vi "NN_Get_Incorrect_Classified_Imgs(GrayScale)_1D.vi"(6 "Test_Data":T2={"Inputs Ref."=variant(refnum<data-value> refnum), "Outputs Ref."=refnum, "Dims_In"=0, "Dataset_Size"=0, "Dims_Out"=0, "Labels"=[], "File Paths"=[]}, 8 "error in (no error)":errorcluster, 10 "Predictions":sgl[][](array[numeric]), 11 "MisClassed_idx":i32[](array[numeric])) -> (0 "error out":errorcluster, 3 "Images(GrayScale)":T1[][](array[typedef])=[[{"image"=array28x28[784 elements], "Truth"=4, "Predicted"=0}, {"image"=array28x28[784 elements], "Truth"=9, "Predicted"=0}, {"image"=array28x28[784 elements], "Truth"=4, "Predicted"=0}, {"image"=array28x28[784 elements], "Truth"=9, "Predicted"=0}, {"image"=array28x28[784 elements], "Truth"=2, "Predicted"=0}, {"image"=array28x28[784 elements], "Truth"=5, "Predicted"=0}, {"image"=array28x28[784 elements], "Truth"=3, "Predicted"=0}, {"image"=array28x28[784 elements], "Truth"=6, "Predicted"=0}, {"image"=array28x28[784 elements], "Truth"=9, "Predicted"=0}, {"image"=array28x28[784 elements], "Truth"=3, "Predicted"=0}], [{"image"=array28x28[784 elements], "Truth"=8, "Predicted"=0}, {"image"=array28x28[784 elements], "Truth"=8, "Predicted"=0}, {"image"=array28x28[784 elements], "Truth"=2, "Predicted"=0}, {"image"=array28x28[784 elements], "Truth"=7, "Predicted"=0}, {"image"=array28x28[784 elements], "Truth"=5, "Predicted"=0}, {"image"=array28x28[784 elements], "Truth"=4, "Predicted"=0}, {"image"=array28x28[784 elements], "Truth"=4, "Predicted"=0}, {"image"=array28x28[784 elements], "Truth"=8, "Predicted"=0}, {"image"=array28x28[784 elements], "Truth"=8, "Predicted"=0}, {"image"=array28x28[784 elements], "Truth"=5, "Predicted"=0}], [{"image"=array28x28[784 elements], "Truth"=5, "Predicted"=0}, {"image"=array28x28[784 elements], "Truth"=6, "Predicted"=0}, {"image"=array28x28[784 elements], "Truth"=7, "Predicted"=0}, {"image"=array28x28[784 elements], "Truth"=4, "Predicted"=0}, {"image"=array28x28[784 elements], "Truth"=3, "Predicted"=0}, {"image"=array28x28[784 elements], "Truth"=7, "Predicted"=0}, {"image"=array28x28[784 elements], "Truth"=6, "Predicted"=0}, {"image"=array28x28[784 elements], "Truth"=9, "Predicted"=0}, {"image"=array28x28[784 elements], "Truth"=2, "Predicted"=0}, {"image"=array28x28[784 elements], "Truth"=7, "Predicted"=0}], [{"image"=array28x28[784 elements], "Truth"=4, "Predicted"=0}, {"image"=array28x28[784 elements], "Truth"=9, "Predicted"=0}, {"image"=array28x28[784 elements], "Truth"=7, "Predicted"=0}, {"image"=array28x28[784 elements], "Truth"=8, "Predicted"=0}, {"image"=array28x28[784 elements], "Truth"=7, "Predicted"=0}, {"image"=array28x28[784 elements], "Truth"=5, "Predicted"=0}, {"image"=array28x28[784 elements], "Truth"=9, "Predicted"=0}, {"image"=array28x28[784 elements], "Truth"=6, "Predicted"=0}, {"image"=array28x28[784 elements], "Truth"=7, "Predicted"=0}, {"image"=array28x28[784 elements], "Truth"=8, "Predicted"=0}], [{"image"=array28x28[784 elements], "Truth"=4, "Predicted"=0}, {"image"=array28x28[784 elements], "Truth"=9, "Predicted"=0}, {"image"=array28x28[784 elements], "Truth"=2, "Predicted"=0}, {"image"=array28x28[784 elements], "Truth"=7, "Predicted"=0}, {"image"=array28x28[784 elements], "Truth"=3, "Predicted"=0}, {"image"=array28x28[784 elements], "Truth"=4, "Predicted"=0}, {"image"=array28x28[784 elements], "Truth"=7, "Predicted"=0}, {"image"=array28x28[784 elements], "Truth"=2, "Predicted"=0}, {"image"=array28x28[784 elements], "Truth"=9, "Predicted"=0}, {"image"=array28x28[784 elements], "Truth"=7, "Predicted"=0}], [{"image"=array28x28[784 elements], "Truth"=0, "Predicted"=0}, {"image"=array28x28[784 elements], "Truth"=7, "Predicted"=0}, {"image"=array28x28[784 elements], "Truth"=7, "Predicted"=0}, {"image"=array28x28[784 elements], "Truth"=5, "Predicted"=0}, {"image"=array28x28[784 elements], "Truth"=4, "Predicted"=0}, {"image"=array28x28[784 elements], "Truth"=3, "Predicted"=0}, {"image"=array28x28[784 elements], "Truth"=6, "Predicted"=0}, {"image"=array28x28[784 elements], "Truth"=4, "Predicted"=0}, {"image"=array28x28[784 elements], "Truth"=6, "Predicted"=0}, {"image"=array28x28[784 elements], "Truth"=1, "Predicted"=0}], [{"image"=array28x28[784 elements], "Truth"=8, "Predicted"=0}, {"image"=array28x28[784 elements], "Truth"=9, "Predicted"=0}, {"image"=array28x28[784 elements], "Truth"=2, "Predicted"=0}, {"image"=array28x28[784 elements], "Truth"=5, "Predicted"=0}, {"image"=array28x28[784 elements], "Truth"=9, "Predicted"=0}, {"image"=array28x28[784 elements], "Truth"=9, "Predicted"=0}, {"image"=array28x28[784 elements], "Truth"=4, "Predicted"=0}, {"image"=array28x28[784 elements], "Truth"=2, "Predicted"=0}, {"image"=array28x28[784 elements], "Truth"=5, "Predicted"=0}, {"image"=array28x28[784 elements], "Truth"=7, "Predicted"=0}], [{"image"=array28x28[784 elements], "Truth"=9, "Predicted"=0}, {"image"=array28x28[784 elements], "Truth"=6, "Predicted"=0}, {"image"=array28x28[784 elements], "Truth"=9, "Predicted"=0}, {"image"=array28x28[784 elements], "Truth"=6, "Predicted"=0}, {"image"=array28x28[784 elements], "Truth"=5, "Predicted"=0}, {"image"=array28x28[784 elements], "Truth"=4, "Predicted"=0}, {"image"=array28x28[784 elements], "Truth"=3, "Predicted"=0}, {"image"=array28x28[784 elements], "Truth"=3, "Predicted"=0}, {"image"=array28x28[784 elements], "Truth"=9, "Predicted"=0}, {"image"=array28x28[784 elements], "Truth"=3, "Predicted"=0}], [{"image"=array28x28[784 elements], "Truth"=6, "Predicted"=0}, {"image"=array28x28[784 elements], "Truth"=9, "Predicted"=0}, {"image"=array28x28[784 elements], "Truth"=1, "Predicted"=0}, {"image"=array28x28[784 elements], "Truth"=5, "Predicted"=0}, {"image"=array28x28[784 elements], "Truth"=4, "Predicted"=0}, {"image"=array28x28[784 elements], "Truth"=4, "Predicted"=0}, {"image"=array28x28[784 elements], "Truth"=6, "Predicted"=0}, {"image"=array28x28[784 elements], "Truth"=9, "Predicted"=0}, {"image"=array28x28[784 elements], "Truth"=6, "Predicted"=0}, {"image"=array28x28[784 elements], "Truth"=5, "Predicted"=0}], [{"image"=array28x28[784 elements], "Truth"=8, "Predicted"=0}, {"image"=array28x28[784 elements], "Truth"=9, "Predicted"=0}, {"image"=array28x28[784 elements], "Truth"=5, "Predicted"=0}, {"image"=array28x28[784 elements], "Truth"=4, "Predicted"=0}, {"image"=array28x28[784 elements], "Truth"=7, "Predicted"=0}, {"image"=array28x28[784 elements], "Truth"=2, "Predicted"=0}, {"image"=array28x28[784 elements], "Truth"=6, "Predicted"=0}, {"image"=array28x28[784 elements], "Truth"=9, "Predicted"=0}, {"image"=array28x28[784 elements], "Truth"=5, "Predicted"=0}, {"image"=array28x28[784 elements], "Truth"=1, "Predicted"=0}], [{"image"=array28x28[784 elements], "Truth"=4, "Predicted"=0}, {"image"=array28x28[784 elements], "Truth"=7, "Predicted"=0}, {"image"=array28x28[784 elements], "Truth"=9, "Predicted"=0}, {"image"=array28x28[784 elements], "Truth"=0, "Predicted"=0}, {"image"=array28x28[784 elements], "Truth"=8, "Predicted"=0}, {"image"=array28x28[784 elements], "Truth"=9, "Predicted"=0}, {"image"=array28x28[784 elements], "Truth"=7, "Predicted"=0}, {"image"=array28x28[784 elements], "Truth"=9, "Predicted"=0}, {"image"=array28x28[784 elements], "Truth"=2, "Predicted"=0}, {"image"=array28x28[784 elements], "Truth"=7, "Predicted"=0}], [{"image"=array28x28[784 elements], "Truth"=2, "Predicted"=0}, {"image"=array28x28[784 elements], "Truth"=5, "Predicted"=0}, {"image"=array28x28[784 elements], "Truth"=2, "Predicted"=0}, {"image"=array28x28[784 elements], "Truth"=7, "Predicted"=0}, {"image"=array28x28[784 elements], "Truth"=3, "Predicted"=0}, {"image"=array28x28[784 elements], "Truth"=8, "Predicted"=0}, {"image"=array28x28[784 elements], "Truth"=6, "Predicted"=0}, {"image"=array28x28[784 elements], "Truth"=8, "Predicted"=0}, {"image"=array28x28[784 elements], "Truth"=8, "Predicted"=0}, {"image"=array28x28[784 elements], "Truth"=8, "Predicted"=0}], [{"image"=array28x28[784 elements], "Truth"=6, "Predicted"=0}, {"image"=array28x28[784 elements], "Truth"=4, "Predicted"=0}, {"image"=array28x28[784 elements], "Truth"=0, "Predicted"=0}, {"image"=array28x28[784 elements], "Truth"=2, "Predicted"=0}, {"image"=array28x28[784 elements], "Truth"=1, "Predicted"=0}, {"image"=array28x28[784 elements], "Truth"=1, "Predicted"=0}, {"image"=array28x28[784 elements], "Truth"=1, "Predicted"=0}, {"image"=array28x28[784 elements], "Truth"=4, "Predicted"=0}, {"image"=array28x28[784 elements], "Truth"=4, "Predicted"=0}, {"image"=array28x28[784 elements], "Truth"=5, "Predicted"=0}], [{"image"=array28x28[784 elements], "Truth"=3, "Predicted"=0}, {"image"=array28x28[784 elements], "Truth"=5, "Predicted"=0}, {"image"=array28x28[784 elements], "Truth"=3, "Predicted"=0}, {"image"=array28x28[784 elements], "Truth"=3, "Predicted"=0}, {"image"=array28x28[784 elements], "Truth"=3, "Predicted"=0}, {"image"=array28x28[784 elements], "Truth"=9, "Predicted"=0}, {"image"=array28x28[784 elements], "Truth"=8, "Predicted"=0}, {"image"=array28x28[784 elements], "Truth"=9, "Predicted"=0}, {"image"=array28x28[784 elements], "Truth"=0, "Predicted"=0}, {"image"=array28x28[784 elements], "Truth"=8, "Predicted"=0}], [{"image"=array28x28[784 elements], "Truth"=1, "Predicted"=0}, {"image"=array28x28[784 elements], "Truth"=6, "Predicted"=0}, {"image"=array28x28[784 elements], "Truth"=0, "Predicted"=0}, {"image"=array28x28[784 elements], "Truth"=2, "Predicted"=0}, {"image"=array28x28[784 elements], "Truth"=6, "Predicted"=0}, {"image"=array28x28[784 elements], "Truth"=0, "Predicted"=0}, {"image"=array28x28[784 elements], "Truth"=8, "Predicted"=0}, {"image"=array28x28[784 elements], "Truth"=8, "Predicted"=0}, {"image"=array28x28[784 elements], "Truth"=7, "Predicted"=0}, {"image"=array28x28[784 elements], "Truth"=7, "Predicted"=0}], [{"image"=array28x28[784 elements], "Truth"=7, "Predicted"=0}, {"image"=array28x28[784 elements], "Truth"=8, "Predicted"=0}, {"image"=array28x28[784 elements], "Truth"=9, "Predicted"=0}, {"image"=array28x28[784 elements], "Truth"=0, "Predicted"=0}, {"image"=array28x28[784 elements], "Truth"=2, "Predicted"=0}, {"image"=array28x28[784 elements], "Truth"=6, "Predicted"=0}, {"image"=array28x28[784 elements], "Truth"=9, "Predicted"=0}, {"image"=array28x28[784 elements], "Truth"=5, "Predicted"=0}, {"image"=array28x28[784 elements], "Truth"=4, "Predicted"=0}, {"image"=array28x28[784 elements], "Truth"=5, "Predicted"=0}], [{"image"=array28x28[784 elements], "Truth"=6, "Predicted"=0}, {"image"=array28x28[784 elements], "Truth"=4, "Predicted"=0}, {"image"=array28x28[784 elements], "Truth"=9, "Predicted"=0}, {"image"=array28x28[784 elements], "Truth"=2, "Predicted"=0}, {"image"=array28x28[784 elements], "Truth"=6, "Predicted"=0}, {"image"=array28x28[784 elements], "Truth"=3, "Predicted"=0}, {"image"=[], "Truth"=0, "Predicted"=0}, {"image"=[], "Truth"=0, "Predicted"=0}, {"image"=[], "Truth"=0, "Predicted"=0}, {"image"=[], "Truth"=0, "Predicted"=0}]])   [LabVIEW 2020]
doc: "Helper VI for analysis.\nReturns Images as intensity graphs with the ground truth and corresponding predictions."
uses:
  <vilib>/Ngene/Deep Learning Toolkit/Toolkit/NN_Data/API/DataSet/DataSet_Types/NN_DataSet(In1D_Out1D).ctl
  <vilib>/Ngene/Deep Learning Toolkit/Toolkit/NN_Data/Controls/DataRef_Types/2D/NN_Data_ref(2D_SGL).ctl
  Controls/Img_GrayScale.ctl
  <vilib>/Ngene/Deep Learning Toolkit/Toolkit/NN_Data/subVIs/Dataset/NN_Variant_to_DVR/2D/NN_Data_Variant_to_DVR(2D_SGL).vi
  <vilib>/Ngene/Deep Learning Toolkit/Toolkit/Deep_Learning_Toolkit_by_Ngene.lvlib
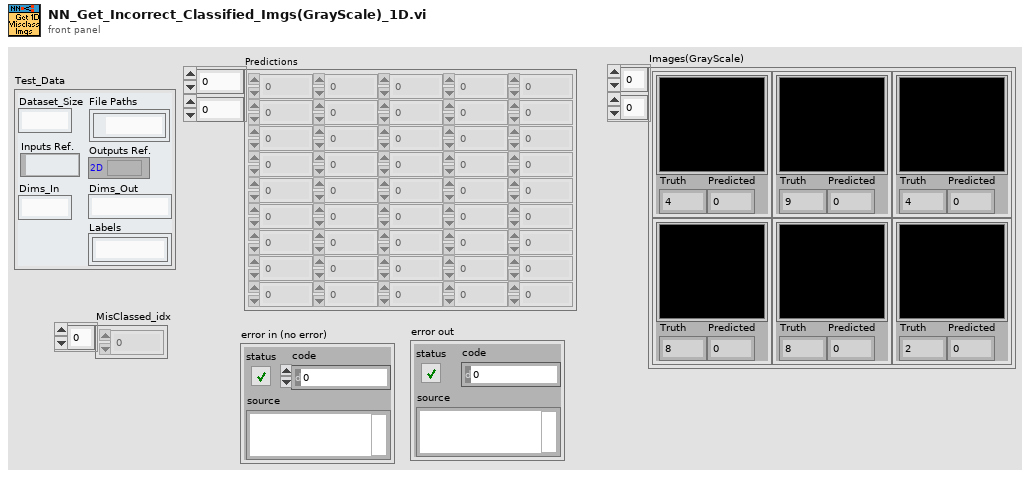
[diagram p1: front panel]
types:
  T1 = typedef "Img_GrayScale.ctl" = cluster{"image":sgl[][], "Truth":i32, "Predicted":i32}
  T2 = typedef "Deep_Learning_Toolkit_by_Ngene.lvlib/NN_DataSet(In1D_Out1D).ctl" = cluster{"Inputs Ref.":variant, "Outputs Ref.":T3, "Dims_In":i32, "Dataset_Size":i32, "Dims_Out":i32, "Labels":string[], "File Paths":path[]}
  T3 = typedef "Deep_Learning_Toolkit_by_Ngene.lvlib/NN_Data_ref(2D_SGL).ctl" = refnum<data-value>
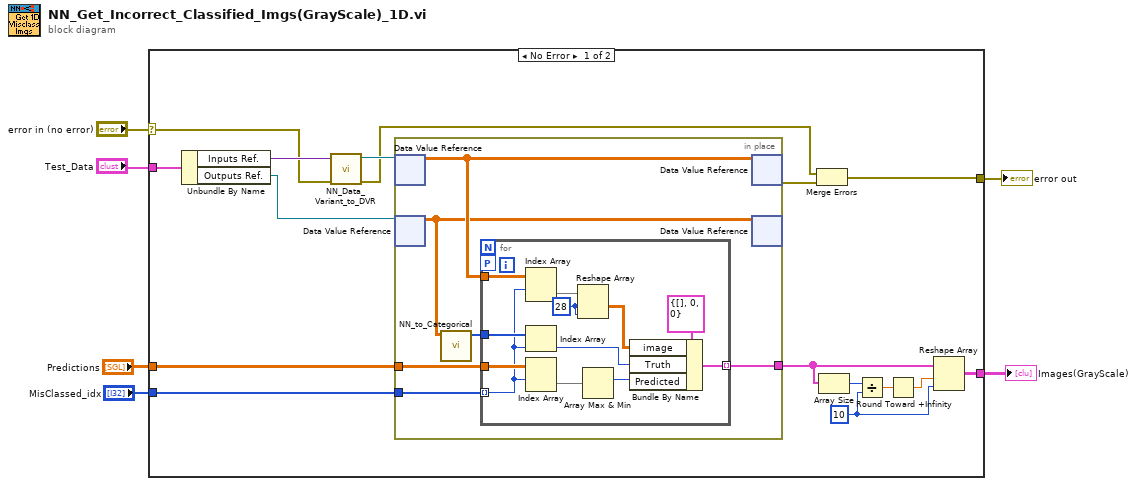
[diagram p0: block diagram]
diagram:
  n1 = case shown="No Error" "error in (no error)" {
    selector: "error in (no error)" -> [w10 w41]
    tunnel: [w13 w41] -> w6
    tunnel: "Test_Data" -> [w18 _]
    tunnel: [w17 _] -> w3
    tunnel: "Predictions" -> [w15 _]
    tunnel: "MisClassed_idx" -> [w14 _]
    frame No Error {
      w19 = 10 ("No_Of_Cols")
      n2 = Unbundle By Name(w18) -> ("Inputs Ref."=w11:variant, "Outputs Ref."=w16:T3)
      n3 = call-poly <vilib>:"NN_Data_Variant_to_DVR.vi"("error in (no error)"=w10, "Inputs Ref."=w11) -> ("error out"=w8:errorcluster, "DVR(2D_SGL)"=w9:T3)  [unwired: 8 in]
      n4 = in-place {
        in-place-border: w14 -> [w28]
        in-place-border: w15 -> [w24]
        in-place-border: [w26] -> w12
        n5 = in-place-dvr #1(w9) -> (w27:sgl[][])  [unwired: 1 out]
        n6 = in-place-dvr #2(w16) -> (w23:sgl[][])  [unwired: 1 out]
        n7 = call <vilib>:"NN_to_Categorical.vi"("Prediction"=w23) -> ("Label_Idx"=w25:i32[])  [unwired: 10 in]
        n8 = for {
          tunnel: w27 -> [w40]
          tunnel: w28 -> [w37] mode=indexing
          workers-P: _ -> [_]
          tunnel: w25 -> [w39]
          tunnel: w24 -> [w38]
          tunnel: [w32] -> w26 mode=indexing
          w29 = 28 ("dimension size")
          n9 = Index Array(array=w40, index (row)=w37) -> (element=w31:sgl[])  [unwired: 1 in]
          n10 = Index Array(array=w39, index=w37) -> (element=w34:i32)
          n11 = Index Array(array=w38, index (row)=w37) -> (element=w33:sgl[])  [unwired: 1 in]
          n12 = Reshape Array(w31, w29, w29) -> (w30:sgl[][])
          n13 = Array Max & Min(array=w33) -> (max index (indices)=w36:i32)  [unwired: 3 out]
          n14 = Bundle By Name(cluster=T1 {"image"=[], "Truth"=0, "Predicted"=0}, "image"=w30, "Truth"=w34, "Predicted"=w36) -> (w32:T1)
        }
        n15 = in-place-dvr #1(w27) -> (w7:errorcluster)  [unwired: 1 out]
        n16 = in-place-dvr #2(w23) -> ()  [unwired: 2 out]
      }
      n17 = Merge Errors(w8, w7) -> (w13:errorcluster)
      n18 = Array Size(array=w12) -> (size(s)=w22:i32)
      n19 = Divide(x=w22, y=w19) -> (x/y=w21:dbl)
      n20 = Round Toward +Infinity(x=w21) -> (ceil(x): smallest int >= x=w20:dbl)
      n21 = Reshape Array(w12, w20, w19) -> (w17:T1[][])
    }
    frame Error {
    }
  }
  "error out" <- w6
  "Images(GrayScale)" <- w3
